vi "LOAD_TCP_CONFIG.vi"() -> (2 "PortNumber":u16=25534, 3 "IP Addr":string="192.168.0.100")   [LabVIEW 2023]
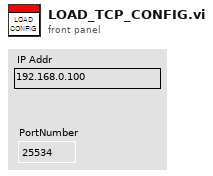
[diagram p1: front panel]
types:
  T1 = enum16{"open", "replace", "create", "open or create", "replace or create", "replace or create with confirmation"}
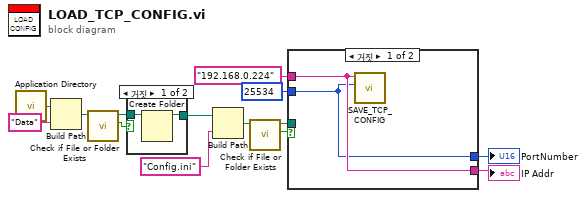
[diagram p0: block diagram]
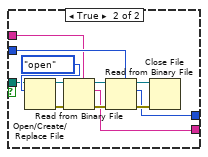
[diagram p3: hidden frame]
diagram:
  n1 = call <vilib>:"Application Directory.vi"() -> ("Application Directory"=w10:path)
  n2 = Build Path(base path=w10, name or relative path="Data" ("이름 또는 상대 경로")) -> (appended path=w12:path)
  n3 = call <vilib>:"Check if File or Folder Exists.vi"("path"=w12) -> ("file or folder exists?"=w13:bool, "dup path"=w14:path)  [unwired: 8 in, 1 out]
  n4 = case shown="거짓" w13 {
    tunnel: w14 -> [w16 w17]
    tunnel: [w15 w17] -> w9
    frame False {
      n5 = Create Folder(path (use dialog)=w16) -> (created path=w15:path)  [unwired: 2 in, 2 out]
    }
    frame True {
    }
  }
  n6 = Build Path(base path=w9, name or relative path="Config.ini" ("이름 또는 상대 경로")) -> (appended path=w8:path)
  n7 = call <vilib>:"Check if File or Folder Exists.vi"("path"=w8) -> ("file or folder exists?"=w5:bool, "dup path"=w6:path)  [unwired: 8 in, 1 out]
  n8 = case shown="거짓" w5 {
    tunnel: w6 -> [_ w23]
    tunnel: u16 25534 ("PortNumber 2") -> [w18 w24]
    tunnel: [w18 w21] -> w3
    tunnel: [w19 w22] -> w2
    tunnel: "192.168.0.224" ("IP Addr 2") -> [w19 w20]
    frame False {
      n9 = call "SAVE_TCP_CONFIG.vi"("PortNumber"=w18, "IP Addr"=w19) -> ()  [unwired: 9 in, 1 out]
    }
    frame True {
      n10 = Open/Create/Replace File(file path (use dialog)=w23, operation (0:open)=T1."open" ("동작(0:open)")) -> (refnum out=w30:refnum<file>, error out=w31:errorcluster)  [unwired: 4 in, 1 out]
      n11 = Read from Binary File(5:w20, 8:w31, 11:w30) -> (0:w27:errorcluster, 2:w22:string, 3:w28:refnum<file>)  [unwired: 3 in, 1 out]
      n12 = Read from Binary File(5:w24, 8:w27, 11:w28) -> (0:w25:errorcluster, 2:w21:u16, 3:w26:refnum<file>)  [unwired: 3 in, 1 out]
      n13 = Close File(refnum=w26, error in=w25) -> ()  [unwired: 2 out]
    }
  }
  "PortNumber" <- w3
  "IP Addr" <- w2
